vi "Set cif_manager_LauncherInfo.vi"(7 "Complete Call (T)":bool=TRUE, 8 "error in (no error)":errorcluster, 10 "package_templatemessage":T1, 11 "gRPCid":T3) -> (0 "error out":errorcluster)   [LabVIEW 2021, in "CIF_Launcher_server.lvlib"]
uses:
  CIF_Launcher_server.lvlib
  <vilib>/gRPC/LabVIEW gRPC Library/Shared/grpcId.ctl
  cif_manager_LauncherInfo.ctl
  cif_manager_LauncherType.ctl
  cif_manager_LauncherInfo_Flat.ctl
  dcc74a39-081a-4bdd-860b-8ed792803c96.vi
  <vilib>/gRPC/LabVIEW gRPC Library/Shared/TranslateGrpcError.vi
  <vilib>/gRPC/LabVIEW gRPC Library/Server API/Server/Get Server DLL Path.vi
  <vilib>/Utility/error.llb/Error Cluster From Error Code.vi
  <vilib>/gRPC/LabVIEW gRPC Library/grpc-lvsupport-release.lvlib
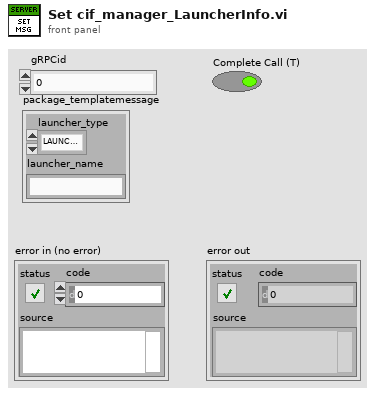
[diagram p1: front panel]
types:
  T1 = typedef "CIF_Launcher_server.lvlib/cif_manager_LauncherInfo.ctl" = cluster{"launcher_type":T2, "launcher_name":string}
  T2 = typedef "CIF_Launcher_server.lvlib/cif_manager_LauncherType.ctl" = enum32{"LAUNCHERTYPE_UNKNOWN", "LAUNCHERTYPE_LABVIEW"}
  T3 = typedef "grpc-lvsupport-release.lvlib/grpcId.ctl" = u64
  T4 = typedef "CIF_Launcher_server.lvlib/cif_manager_LauncherInfo_Flat.ctl" = cluster{"launcher_type":T2, "launcher_name":string}
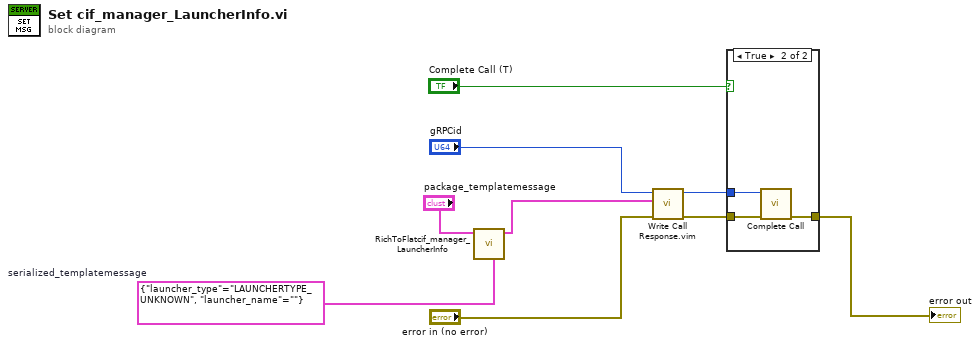
[diagram p0: block diagram]
diagram:
  w2 = T4 {"launcher_type"=enum."LAUNCHERTYPE_UNKNOWN", "launcher_name"=""}  # serialized_templatemessage
  n1 = call "RichToFlatcif_manager_LauncherInfo.vi"("OutputClusterType"=w2, "InputCluster"="package_templatemessage") -> ("OutputCluster"=w1:T4)  [unwired: 9 in]
  n2 = call "Write Call Response.vim"("error in"="error in (no error)", "Response Data"=w1, "gRPCid in"="gRPCid") -> ("error out"=w6:errorcluster, "gRPCid out"=w7:T3)  [unwired: 7 in]
  n3 = case shown="True" "Complete Call (T)" {
    tunnel: [w10 w13] -> w9
    tunnel: w7 -> [_ w12]
    tunnel: w6 -> [w10 w11]
    frame False {
    }
    frame True {
      n4 = call <vilib>:"Complete Call.vi"("gRPCid"=w12, "error in"=w11) -> ("error out"=w13:errorcluster)  [unwired: 8 in]
    }
  }
  "error out" <- w9
